vi "ReadStatusAllPumps.vi"(0 "object in":refnum<class "CetoniPump.lvclass">, 5 "error in (no error)":errorcluster) -> (14 "object out":refnum<class "CetoniPump.lvclass">, 16 "Array":T1(array[cluster]), 19 "error out":errorcluster)   [LabVIEW 2021, in "CetoniPump.lvclass"]
uses:
  CetoniPump.lvclass
  CetoniPump.lvclass/CetoniPump.ctl
  Users/olaja/AppData/Local/CETONI_SDK/lib/labview/labbCAN_Pump_API/labbCAN_Pump_API.lvlib
panel:
  in  "Cluster":T2
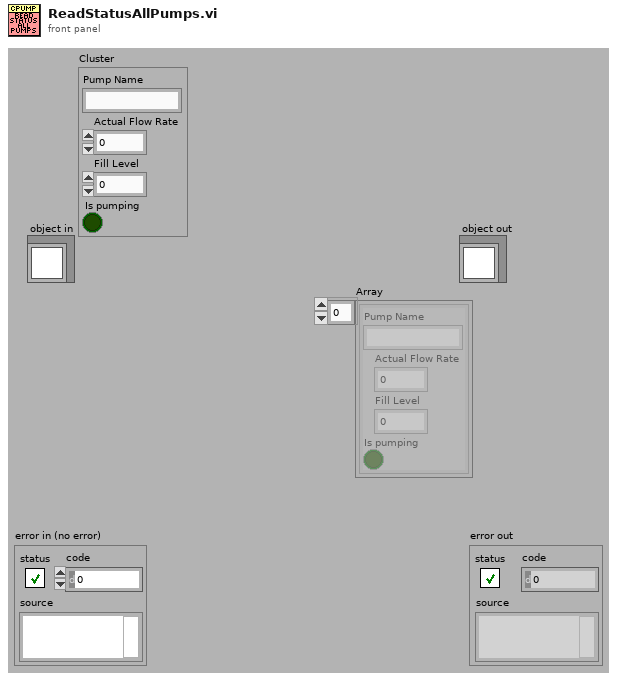
[diagram p1: front panel]
types:
  T1 = cluster{"Pump Name":string, "Actual Flow Rate":dbl, "Fill Level":dbl, "Is pumping":bool}[]
  T2 = cluster{"Pump Name":string, "Actual Flow Rate":dbl, "Fill Level":dbl, "Is pumping":bool}
  T3 = cluster{"Pump Handle":i64, "Pump Name":string, "Maximum Volume":dbl, "Maximum Flow Rate":dbl, "Flow Rate":dbl, "Target Level":dbl}[]
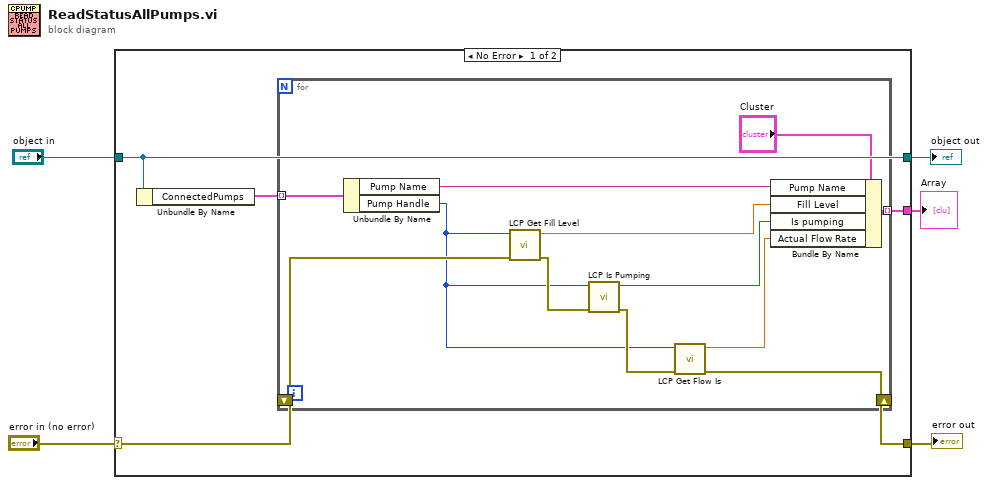
[diagram p0: block diagram]
diagram:
  n1 = case shown="No Error" "error in (no error)" {
    selector: "error in (no error)" -> [w9 w24]
    tunnel: [w8 w24] -> w4
    tunnel: [w10 w23] -> w2
    tunnel: "object in" -> [w10 w23]
    tunnel: [w6 _] -> w1
    frame No Error {
      n2 = Unbundle By Name(w10) -> ("ConnectedPumps"=w7:T3)
      n3 = for {
        shift-right: [w21] -> w8
        shift-left: w9 -> [w22]
        tunnel: w7 -> [w14] mode=indexing
        tunnel: [w11] -> w6 mode=indexing
        n4 = Unbundle By Name(w14) -> ("Pump Name"=w13:string, "Pump Handle"=w12:i64)
        n5 = call "LCP Get Fill Level.vi"("error in (no error)"=w22, "Pump Handle"=w12) -> ("error out"=w20:errorcluster, "Fill Level"=w17:dbl)  [unwired: 8 in]
        n6 = call "LCP Is Pumping.vi"("error in (no error)"=w20, "Pump Handle"=w12) -> ("error out"=w19:errorcluster, "Is pumping"=w16:bool)  [unwired: 8 in]
        n7 = call "LCP Get Flow Is.vi"("error in (no error)"=w19, "Pump Handle"=w12) -> ("error out"=w21:errorcluster, "Actual Flow Rate"=w15:dbl)  [unwired: 8 in]
        n8 = Bundle By Name(cluster="Cluster", "Pump Name"=w13, "Fill Level"=w17, "Is pumping"=w16, "Actual Flow Rate"=w15) -> (w11:T2)
      }
    }
    frame Error {
    }
  }
  "error out" <- w4
  "object out" <- w2
  "Array" <- w1
